vi "sevensegment(SubVI).vi"(11 "Numeric":i32) -> (0 "Boolean 5":bool, 1 "Boolean 6":bool, 2 "Boolean 2":bool, 3 "Boolean 7":bool, 4 "Boolean 4":bool, 5 "Boolean 8":bool, 6 "Boolean 3":bool, 7 "Boolean":bool)   [LabVIEW 2017]
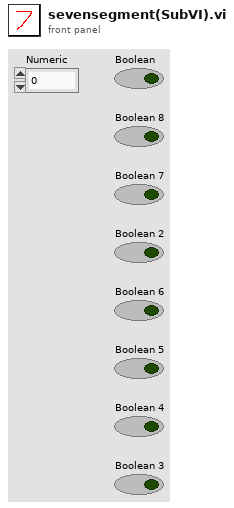
[diagram p1: front panel]
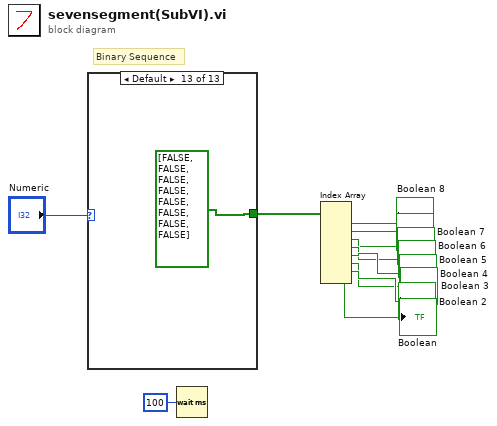
[diagram p0: block diagram]
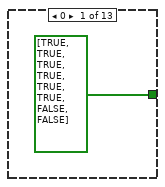
[diagram p2: hidden frame]
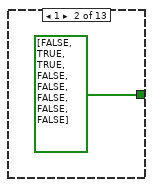
[diagram p3: hidden frame]
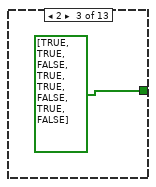
[diagram p4: hidden frame]
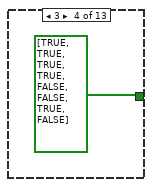
[diagram p5: hidden frame]
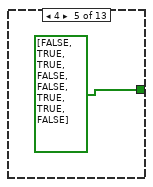
[diagram p6: hidden frame]
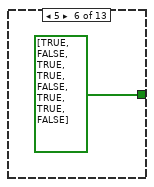
[diagram p7: hidden frame]
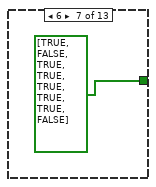
[diagram p8: hidden frame]
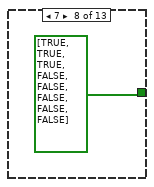
[diagram p9: hidden frame]
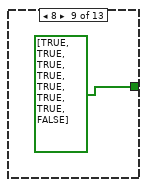
[diagram p10: hidden frame]
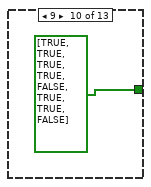
[diagram p11: hidden frame]
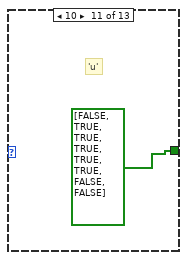
[diagram p12: hidden frame]
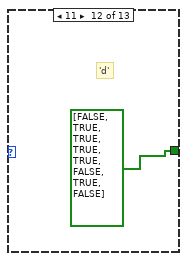
[diagram p13: hidden frame]
diagram:
  # "Binary Sequence"
  n1 = case shown="Default" "Numeric" {
    tunnel: [bool[] [TRUE, TRUE, TRUE, TRUE, TRUE, TRUE, FALSE, FALSE] bool[] [FALSE, TRUE, TRUE, FALSE, FALSE, FALSE, FALSE, FALSE] bool[] [TRUE, TRUE, FALSE, TRUE, TRUE, FALSE, TRUE, FALSE] bool[] [TRUE, TRUE, TRUE, TRUE, FALSE, FALSE, TRUE, FALSE] bool[] [FALSE, TRUE, TRUE, FALSE, FALSE, TRUE, TRUE, FALSE] bool[] [TRUE, FALSE, TRUE, TRUE, FALSE, TRUE, TRUE, FALSE] bool[] [TRUE, FALSE, TRUE, TRUE, TRUE, TRUE, TRUE, FALSE] bool[] [TRUE, TRUE, TRUE, FALSE, FALSE, FALSE, FALSE, FALSE] bool[] [TRUE, TRUE, TRUE, TRUE, TRUE, TRUE, TRUE, FALSE] bool[] [TRUE, TRUE, TRUE, TRUE, FALSE, TRUE, TRUE, FALSE] bool[] [FALSE, TRUE, TRUE, TRUE, TRUE, TRUE, FALSE, FALSE] bool[] [FALSE, TRUE, TRUE, TRUE, TRUE, FALSE, TRUE, FALSE] bool[] [FALSE, FALSE, FALSE, FALSE, FALSE, FALSE, FALSE, FALSE]] -> w2
    frame 0 {
    }
    frame 1 {
    }
    frame 2 {
    }
    frame 3 {
    }
    frame 4 {
    }
    frame 5 {
    }
    frame 6 {
    }
    frame 7 {
    }
    frame 8 {
    }
    frame 9 {
    }
    frame 10 {
      # "'u'"
    }
    frame 11 {
      # "'d'"
    }
    frame Default {
    }
  }
  n2 = Wait (ms)(milliseconds to wait=u32 100) -> ()  [unwired: 1 out]
  n3 = Index Array(array=w2) -> (element #1=→"Boolean 8":bool, element #2=→"Boolean 7":bool, element #3=→"Boolean 6":bool, element #4=→"Boolean 5":bool, element #5=→"Boolean 4":bool, element #6=→"Boolean 3":bool, element #7=→"Boolean 2":bool, element #8=→"Boolean":bool)  [unwired: 8 in]
